vi "Agilent VNA Read Sweep Type.vi"(6 "Channel":i8=1 min=1 max=99 step=1, 7 "Agilent VNA":T1, 8 "error in (no error)":errorcluster, 11 "VISA Resource Name":refnum<visa-resource-name>) -> (0 "error out":errorcluster, 2 "Sweep Type":T2, 3 "dup VISA Resource Name":refnum<visa-resource-name>)   [LabVIEW 2011]
doc: "This VI for the HP 8753 is used to read the sweep type.\n\n0 LINEAR FREQ\n1 LOG FREQ\n2 LIST FREQ\n3 CW TIME\n4 POWER SWEEP"
uses:
  TypeDefs/Agilent VNA Sweep Type.ctl
  TypeDefs/Agilent VNA Instrument Info.ctl
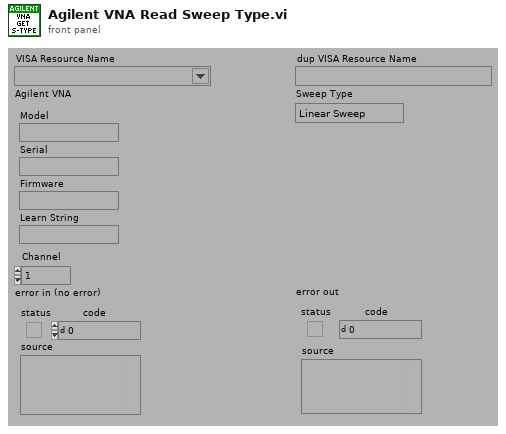
[diagram p1: front panel]
types:
  T1 = typedef "Agilent VNA Instrument Info.ctl" = cluster{"Model":string, "Serial":string, "Firmware":string, "Learn String":string}
  T2 = typedef "Agilent VNA Sweep Type.ctl" = enum32{"Linear Sweep", "Logarithmic Sweep", "Frequency List", "CW Time Sweep", "Power Sweep"}
  T3 = typedef "Agilent VNA Model.ctl" = enum16{"Not Supported", "8510X", "8719X", "8720X", "8722X", "8753X", "ENA", "PNA", "Field Fox"}
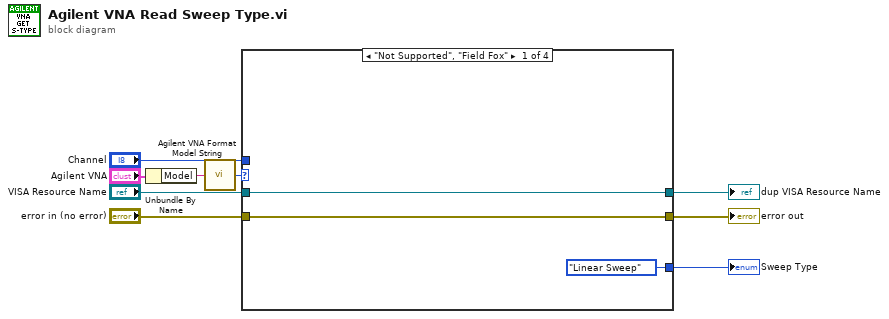
[diagram p0: block diagram]
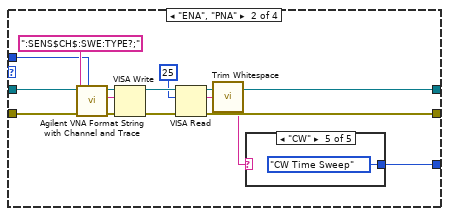
[diagram p2: hidden frame]
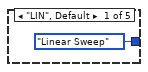
[diagram p3: hidden frame]
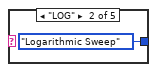
[diagram p4: hidden frame]
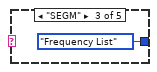
[diagram p5: hidden frame]
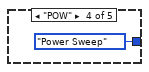
[diagram p6: hidden frame]
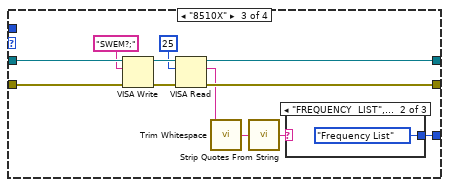
[diagram p7: hidden frame]
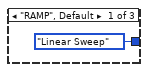
[diagram p8: hidden frame]
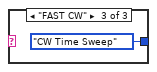
[diagram p9: hidden frame]
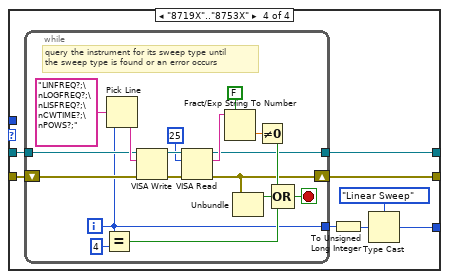
[diagram p10: hidden frame]
diagram:
  n1 = Unbundle By Name("Agilent VNA") -> ("Model"=w1:string)
  n2 = call "Agilent VNA Format Model String.vi"("Model"=w1) -> ("Model"=w4:T3)
  n3 = case shown="\"Not Supported\", \"Field Fox\"" w4 {
    tunnel: "VISA Resource Name" -> [w12 w21 w38 w53]
    tunnel: "error in (no error)" -> [w11 w25 w42 w52]
    tunnel: [w11 w24 w41 w51] -> w8
    tunnel: [Agilent_VNA_Sweep_Type."Linear Sweep" ("sweep type") w18 w35 w49] -> w7
    tunnel: [w12 w19 w36 w46] -> w5
    tunnel: "Channel" -> [_ w13 _ _]
    frame "Not Supported", "Field Fox" {
    }
    frame "ENA", "PNA" {
      n4 = call "Agilent VNA Format String with Channel and Trace.vi"("Channel"=w13, "String"=":SENS$CH$:SWE:TYPE?;") -> ("String Out"=w14:string)  [unwired: 1 in, 6 out]
      n5 = VISA Write(VISA resource name=w21, write buffer=w14, error in (no error)=w25) -> (VISA resource name out=w22:refnum<visa-resource-name>, error out=w23:errorcluster)  [unwired: 1 out]
      n6 = VISA Read(VISA resource name=w22, byte count=u32 25, error in (no error)=w23) -> (VISA resource name out=w19:refnum<visa-resource-name>, read buffer=w17:string, error out=w24:errorcluster)  [unwired: 1 out]
      n7 = call <vilib>:"Trim Whitespace.vi"("string"=w17) -> ("trimmed string"=w16:string)  [unwired: 1 in]
      n8 = case shown="\"CW\"" w16 {
        tunnel: [Agilent_VNA_Sweep_Type."Linear Sweep" ("sweep type") Agilent_VNA_Sweep_Type."Logarithmic Sweep" ("sweep type") Agilent_VNA_Sweep_Type."Frequency List" ("sweep type") Agilent_VNA_Sweep_Type."Power Sweep" ("sweep type") Agilent_VNA_Sweep_Type."CW Time Sweep" ("sweep type")] -> w18
        frame "LIN", Default {
        }
        frame "LOG" {
        }
        frame "SEGM" {
        }
        frame "POW" {
        }
        frame "CW" {
        }
      }
    }
    frame "8510X" {
      n9 = VISA Write(VISA resource name=w38, write buffer="SWEM?;", error in (no error)=w42) -> (VISA resource name out=w39:refnum<visa-resource-name>, error out=w40:errorcluster)  [unwired: 1 out]
      n10 = VISA Read(VISA resource name=w39, byte count=u32 25, error in (no error)=w40) -> (VISA resource name out=w36:refnum<visa-resource-name>, read buffer=w34:string, error out=w41:errorcluster)  [unwired: 1 out]
      n11 = call <vilib>:"Trim Whitespace.vi"("string"=w34) -> ("trimmed string"=w32:string)  [unwired: 1 in]
      n12 = call "Strip Quotes From String.vi"("String In"=w32) -> ("Trimmed String"=w31:string)
      n13 = case shown="\"FREQUENCY  LIST\", \"SINGLE POINT\", \"STEP\"" w31 {
        tunnel: [Agilent_VNA_Sweep_Type."Linear Sweep" ("sweep type") Agilent_VNA_Sweep_Type."Frequency List" ("sweep type") Agilent_VNA_Sweep_Type."CW Time Sweep" ("sweep type")] -> w35
        frame "RAMP", Default {
        }
        frame "FREQUENCY  LIST", "SINGLE POINT", "STEP" {
        }
        frame "FAST CW" {
        }
      }
    }
    frame "8719X".."8753X" {
      n14 = while {
        tunnel: w53 -> [w64]
        shift-right: [w57] -> w51
        shift-left: w52 -> [w58]
        tunnel: [w55] -> w47
        tunnel: [w54] -> w46
        i -> [w55]
        stop <- w65 stop-if-true
        # "query the instrument for its sweep type until\nthe sweep type is found or an error occurs"
        n15 = Equal?(x=w55, y=4) -> (x = y?=w56:bool)
        n16 = Pick Line(multi-line string="LINFREQ?;\nLOGFREQ?;\nLISFREQ?;\nCWTIME?;\nPOWS?;", line index=w55) -> (output string=w70:string)  [unwired: 1 out]
        n17 = VISA Write(VISA resource name=w64, write buffer=w70, error in (no error)=w58) -> (VISA resource name out=w63:refnum<visa-resource-name>, error out=w69:errorcluster)  [unwired: 1 out]
        n18 = VISA Read(VISA resource name=w63, byte count=u32 25, error in (no error)=w69) -> (VISA resource name out=w54:refnum<visa-resource-name>, read buffer=w68:string, error out=w57:errorcluster)  [unwired: 1 out]
        n19 = Fract/Exp String To Number(use system decimal point (T)=FALSE, string=w68) -> (number=w67:dbl)  [unwired: 3 out]
        n20 = Unbundle(w57) -> ("status"=w59:bool)  [unwired: 2 out]
        n21 = Not Equal To 0?(x=w67) -> (x != 0?=w66:bool)
        n22 = Compound Arithmetic op=OR(w66, w59, w56) -> (w65:bool)
      }
      n23 = To Unsigned Long Integer(number=w47) -> (unsigned 32bit integer=w48:u32)
      n24 = Type Cast(type=Agilent_VNA_Sweep_Type."Linear Sweep" ("sweep type"), x=w48) -> (*(type *) &x=w49:T2)
    }
  }
  "Sweep Type" <- w7
  "dup VISA Resource Name" <- w5
  "error out" <- w8
